vi "Get String Data.vi"(11 "ERD_Always Show":T1) -> (3 "ERD String":string[][](array[string]))   [LabVIEW 2014]
uses:
  GitHome/Tools/Laundry/Washer Soft Load Box/type defs/ERD_Always_Show.ctl
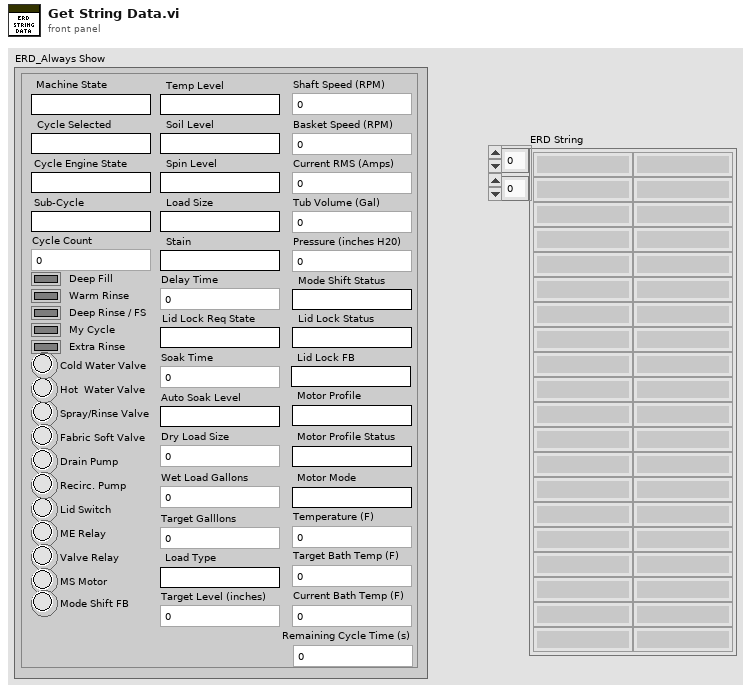
[diagram p1: front panel]
types:
  T1 = typedef "ERD_Always_Show.ctl" = cluster{"Basket Speed (RPM)":u16, "Machine State":string, "Tub Volume (Gal)":dbl, "Pressure (inches H20)":dbl, "Lid Switch ":bool, "Current RMS (Amps)":dbl, "Cycle Selected":string, "Lid Lock Status":string, "Mode Shift Status":string, "Spray/Rinse Valve":bool, "Fabric Soft Valve":bool, "Drain Pump":bool, "Recirc. Pump":bool, "Cycle Engine State":string, "Hot  Water Valve":bool, "Cold Water Valve":bool, "Motor Profile":string, "Motor Profile Status":string, "Motor Mode":string, "ME Relay":bool, "Cycle Count":u32, "Deep Rinse / FS":bool, "My Cycle":bool, "Soil Level":string, "Spin Level":string, "Stain":string, "Temp Level":string, "Load Size":string, "Delay Time":u16, "Soak Time":u16, "Deep Fill":bool, "Warm Rinse":bool, "Auto Soak Level":string, "Extra Rinse":bool, "Wet Load Gallons":dbl, "Target Galllons":dbl, "Sub-Cycle":string, "Load Type":string, "Target Level (inches)":u32, "Valve Relay":bool, "Dry Load Size":dbl, "Shaft Speed (RPM) ":u16, "MS Motor":bool, "Mode Shift FB":bool, "Target Bath Temp (F)":dbl, "Temperature (F)":dbl, "Current Bath Temp (F)":dbl, "Lid Lock FB":string, "Lid Lock Req State":string, "Remaining Cycle Time (s)":dbl}
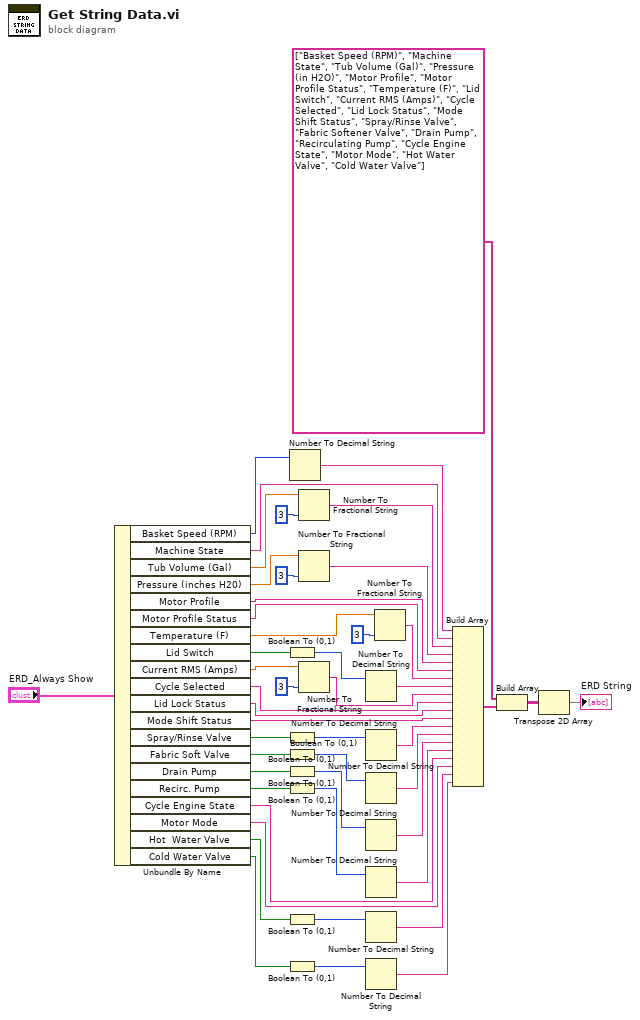
[diagram p0: block diagram]
diagram:
  n1 = Unbundle By Name("ERD_Always Show") -> ("Basket Speed (RPM)"=w47:u16, "Machine State"=w45:string, "Tub Volume (Gal)"=w44:dbl, "Pressure (inches H20)"=w40:dbl, "Motor Profile"=w38:string, "Motor Profile Status"=w37:string, "Temperature (F)"=w35:dbl, "Lid Switch"=w32:bool, "Current RMS (Amps)"=w29:dbl, "Cycle Selected"=w27:string, "Lid Lock Status"=w26:string, "Mode Shift Status"=w25:string, "Spray/Rinse Valve"=w23:bool, "Fabric Soft Valve"=w20:bool, "Drain Pump"=w17:bool, "Recirc. Pump"=w14:bool, "Cycle Engine State"=w11:string, "Motor Mode"=w10:string, "Hot  Water Valve"=w9:bool, "Cold Water Valve"=w6:bool)
  n2 = Boolean To (0,1)(Boolean=w32) -> (0, 1=w33:i16)
  n3 = Boolean To (0,1)(Boolean=w23) -> (0, 1=w24:i16)
  n4 = Boolean To (0,1)(Boolean=w20) -> (0, 1=w21:i16)
  n5 = Boolean To (0,1)(Boolean=w17) -> (0, 1=w18:i16)
  n6 = Boolean To (0,1)(Boolean=w14) -> (0, 1=w15:i16)
  n7 = Boolean To (0,1)(Boolean=w9) -> (0, 1=w12:i16)
  n8 = Boolean To (0,1)(Boolean=w6) -> (0, 1=w7:i16)
  n9 = Number To Decimal String(number=w47) -> (decimal integer string=w46:string)  [unwired: 1 in]
  n10 = Number To Fractional String(number=w44, precision (6)=i16 3) -> (F-format string=w42:string)  [unwired: 2 in]
  n11 = Number To Fractional String(number=w40, precision (6)=i16 3) -> (F-format string=w39:string)  [unwired: 2 in]
  n12 = Number To Fractional String(number=w29, precision (6)=i16 3) -> (F-format string=w28:string)  [unwired: 2 in]
  n13 = Number To Decimal String(number=w33) -> (decimal integer string=w31:string)  [unwired: 1 in]
  n14 = Number To Decimal String(number=w24) -> (decimal integer string=w22:string)  [unwired: 1 in]
  n15 = Number To Decimal String(number=w21) -> (decimal integer string=w19:string)  [unwired: 1 in]
  n16 = Number To Decimal String(number=w18) -> (decimal integer string=w16:string)  [unwired: 1 in]
  n17 = Number To Decimal String(number=w15) -> (decimal integer string=w13:string)  [unwired: 1 in]
  n18 = Number To Decimal String(number=w12) -> (decimal integer string=w8:string)  [unwired: 1 in]
  n19 = Number To Decimal String(number=w7) -> (decimal integer string=w5:string)  [unwired: 1 in]
  n20 = Number To Fractional String(number=w35, precision (6)=i16 3) -> (F-format string=w34:string)  [unwired: 2 in]
  n21 = Build Array(w46, w45, w42, w39, w38, w37, w34, w31, w28, w27, w26, w25, w22, w19, w16, w13, w11, w10, w8, w5) -> (w4:string[])
  n22 = Build Array(string[] ["Basket Speed (RPM)", "Machine State", "Tub Volume (Gal)", "Pressure (in H2O)", "Motor Profile", "Motor Profile Status", "Temperature (F)", "Lid Switch", "Current RMS (Amps)", "Cycle Selected", "Lid Lock Status", "Mode Shift Status", "Spray/Rinse Valve", "Fabric Softener Valve", "Drain Pump", "Recirculating Pump", "Cycle Engine State", "Motor Mode", "Hot Water Valve", "Cold Water Valve"], w4) -> (w2:string[][])
  n23 = Transpose 2D Array(2D array=w2) -> (transposed array=→"ERD String":string[][])
